vi "创建保存文件.vi"(11 "日期/时间字符串":string) -> (3 "路径":path)   [LabVIEW 2011]
uses:
  Global System.vi
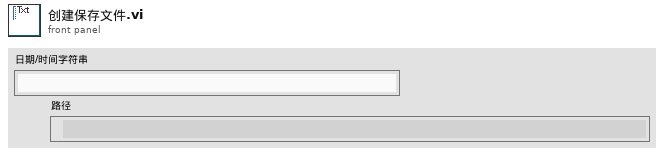
[diagram p1: front panel]
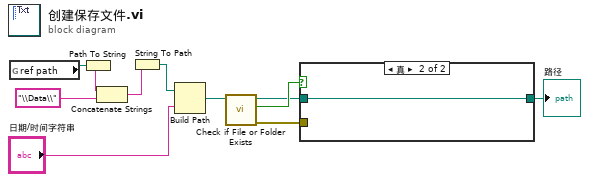
[diagram p0: block diagram]
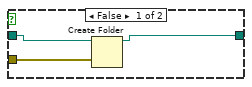
[diagram p2: hidden frame]
diagram:
  n1 = global read "Global System.vi" "ref path"() -> (w7:path)
  n2 = Path To String(path=w7) -> (string=w6:string)
  n3 = Concatenate Strings(w6, "\\Data\\") -> (w4:string)
  n4 = String To Path(string=w4) -> (path=w3:path)
  n5 = Build Path(base path=w3, name or relative path="日期/时间字符串") -> (appended path=w11:path)
  n6 = call <vilib>:"Check if File or Folder Exists.vi"("path"=w11) -> ("error out"=w8:errorcluster, "file or folder exists?"=w10:bool, "dup path"=w9:path)  [unwired: 8 in]
  n7 = case shown="真" w10 {
    tunnel: [w13 w15] -> w1
    tunnel: w9 -> [w14 w15]
    tunnel: w8 -> [w12 _]
    frame False {
      n8 = Create Folder(path (use dialog)=w14, error in=w12) -> (created path=w13:path)  [unwired: 1 in, 2 out]
    }
    frame True {
    }
  }
  "路径" <- w1
